vi "rosinterface-1.vi"() -> ()   [LabVIEW 2016]
uses:
  <userlib>/ROS for LabVIEW Software/ROS/Code/SubVIs/_ROSControl.ctl
  <userlib>/ROS for LabVIEW Software/ROS/Code/SubVIs/_ROSDirection.ctl
  <userlib>/ROS for LabVIEW Software/ROS/Code/Console/Servers/ServerSubs/TopicDef.ctl
  <userlib>/ROS for LabVIEW Software/ROS/MessageBuilding/std_msgs/subs/stringScalar.vi
  <userlib>/ROS for LabVIEW Software/ROS/MessageParsing/std_msgs/subs/parse_string_scalar.vi
panel:
  out "ROS out 2":T1={"topic port"=0, "Node"="", "topic"="", "type"="", "node port"=0, "error "={"status"=FALSE, "code"=0, "source"=""}, "Direction"=enum."Node", "Update (ms)"=1, "FIFO size"=1}
  in  "table 6":bool
  in  "table 5":bool
  in  "table 4":bool
  in  "table 3":bool
  in  "table2":bool
  in  "table 1":bool
  out "ROS out":T1={"topic port"=0, "Node"="", "topic"="", "type"="", "node port"=0, "error "={"status"=FALSE, "code"=0, "source"=""}, "Direction"=enum."Node", "Update (ms)"=1, "FIFO size"=1}
  in  "stop":bool
  out "Table  5":bool
  out "Table  4":bool
  out "Table  3":bool
  out "Table  2":bool
  out "Table 1":bool
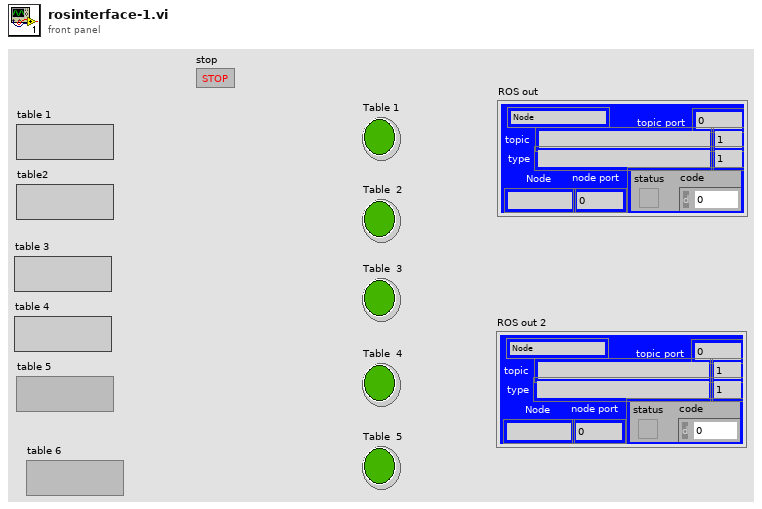
[diagram p1: front panel]
types:
  T1 = typedef "_ROSControl.ctl" = cluster{"topic port":u16, "Node":string, "topic":string, "type":string, "node port":u16, "error ":errorcluster, "Direction":T2, "Update (ms)":u16, "FIFO size":u16}
  T2 = typedef "_ROSDirection.ctl" = enum16{"Node", "Publisher", "Subscriber", "ServiceClient", "ServiceProvider"}
  T3 = typedef "TopicDef.ctl" = cluster{"Topic":string, "Type":string, "Action":T2, "Update (ms)":u16, "queue size":u16}
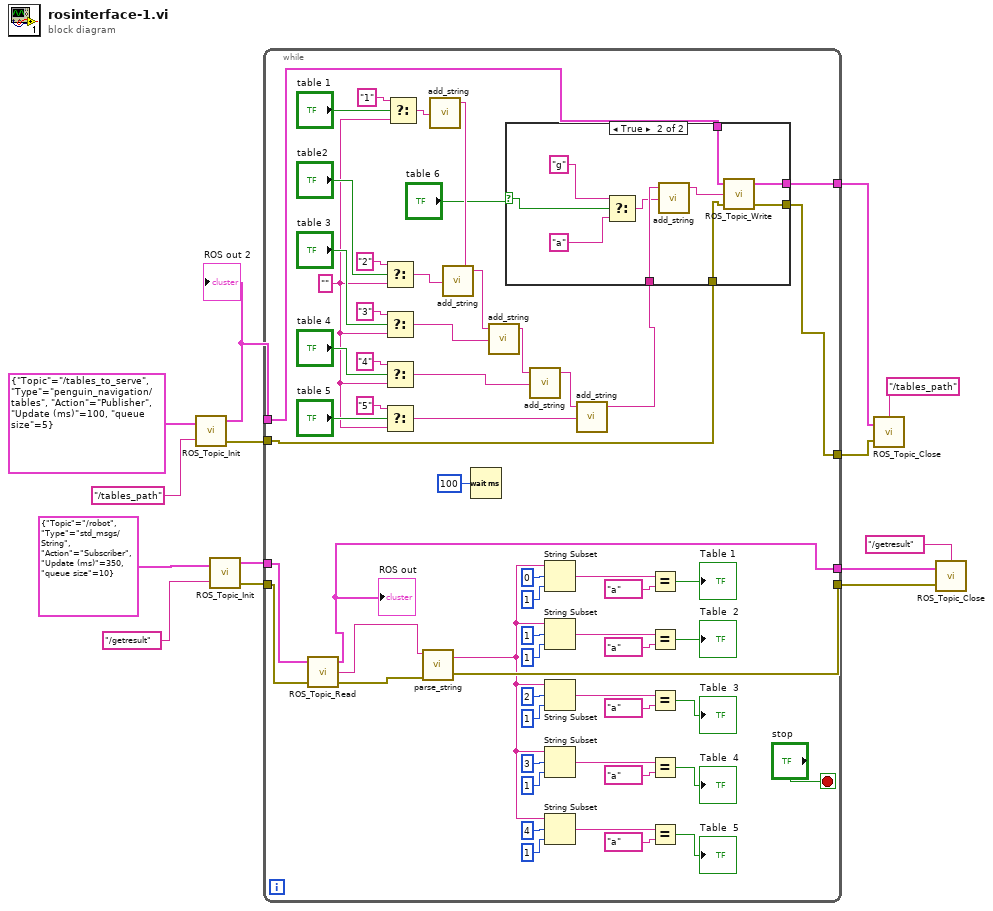
[diagram p0: block diagram]
diagram:
  n1 = call <userlib>:"ROS_Topic_Init.vi"("Definitions"=T3 {"Topic"="/tables_to_serve", "Type"="penguin_navigation/tables", "Action"=enum."Publisher", "Update (ms)"=100, "queue size"=5}, "node"="/tables_path") -> ("ROS out"=w8:T1, "error out"=w7:errorcluster)  [unwired: 1 in]
  "ROS out 2" <- w8
  n2 = call <userlib>:"ROS_Topic_Init.vi"("Definitions"=T3 {"Topic"="/robot", "Type"="std_msgs/String", "Action"=enum."Subscriber", "Update (ms)"=350, "queue size"=10}, "node"="/getresult") -> ("ROS out"=w4:T1, "error out"=w3:errorcluster)  [unwired: 1 in]
  n3 = while {
    tunnel: w4 -> [w28]
    tunnel: [w26] -> w13
    tunnel: w3 -> [w27]
    tunnel: [w74] -> w12
    tunnel: w8 -> [w19]
    tunnel: w7 -> [w18]
    tunnel: [w17] -> w2
    tunnel: [w16] -> w1
    stop <- "stop" stop-if-true
    w61 = "" ("t")
    n4 = call <userlib>:"ROS_Topic_Read.vi"("error in (no error)"=w27, "ROS in"=w28) -> ("error out"=w24:errorcluster, "Reply"=w25:string, "ROS out"=w26:T1)  [unwired: 1 in]
    "ROS out" <- w26
    n5 = Select(t="2", s="table2", f=w61) -> (s? t:f=w69:string)
    n6 = Select(t="3", s="table 3", f=w61) -> (s? t:f=w70:string)
    n7 = Select(t="4", s="table 4", f=w61) -> (s? t:f=w71:string)
    n8 = Select(t="5", s="table 5", f=w61) -> (s? t:f=w72:string)
    n9 = Select(t="1", s="table 1", f=w61) -> (s? t:f=w23:string)
    n10 = call-poly <userlib>:"parse_string.vi"("error in"=w24, "msg in"=w25) -> ("error out"=w74:errorcluster, "string"=w31:string)  [unwired: 3 in, 1 out]
    n11 = call-poly <userlib>:"add_string.vi"("String"=w23) -> ("msg out"=w22:string)  [unwired: 4 in]
    n12 = call-poly <userlib>:"add_string.vi"("String"=w69, "msg in"=w22) -> ("msg out"=w68:string)  [unwired: 3 in]
    n13 = Wait (ms)(milliseconds to wait=u32 100) -> ()  [unwired: 1 out]
    n14 = call-poly <userlib>:"add_string.vi"("String"=w70, "msg in"=w68) -> ("msg out"=w67:string)  [unwired: 3 in]
    n15 = call-poly <userlib>:"add_string.vi"("String"=w71, "msg in"=w67) -> ("msg out"=w73:string)  [unwired: 3 in]
    n16 = String Subset(string=w31, offset (0)=0, length (rest)=1 ("offset (0)")) -> (substring=w45:string)
    n17 = String Subset(string=w31, offset (0)=1, length (rest)=1 ("offset (0)")) -> (substring=w44:string)
    n18 = String Subset(string=w31, offset (0)=2, length (rest)=1 ("offset (0)")) -> (substring=w43:string)
    n19 = String Subset(string=w31, offset (0)=3, length (rest)=1 ("offset (0)")) -> (substring=w42:string)
    n20 = String Subset(string=w31, offset (0)=4, length (rest)=1 ("offset (0)")) -> (substring=w41:string)
    n21 = call-poly <userlib>:"add_string.vi"("String"=w72, "msg in"=w73) -> ("msg out"=w21:string)  [unwired: 3 in]
    n22 = case shown="True" "table 6" {
      selector: "table 6" -> [_ w80]
      tunnel: w21 -> [_ w82]
      tunnel: w19 -> [_ w78]
      tunnel: w18 -> [_ w77]
      tunnel: [_ w76] -> w17
      tunnel: [_ w75] -> w16
      frame False {
      }
      frame True {
        n23 = Select(t="g", s=w80, f="a") -> (s? t:f=w81:string)
        n24 = call-poly <userlib>:"add_string.vi"("String"=w81, "msg in"=w82) -> ("msg out"=w79:string)  [unwired: 3 in]
        n25 = call <userlib>:"ROS_Topic_Write.vi"("error in (no error)"=w77, "Msg in"=w79, "ROS in"=w78) -> ("error out"=w76:errorcluster, "ROS out"=w75:T1)  [unwired: 1 in]
      }
    }
    n26 = Equal?(x=w45, y="a") -> (x = y?=→"Table 1":bool)
    n27 = Equal?(x=w44, y="a") -> (x = y?=→"Table  2":bool)
    n28 = Equal?(x=w43, y="a") -> (x = y?=→"Table  3":bool)
    n29 = Equal?(x=w42, y="a") -> (x = y?=→"Table  4":bool)
    n30 = Equal?(x=w41, y="a") -> (x = y?=→"Table  5":bool)
  }
  n31 = call <userlib>:"ROS_Topic_Close.vi"("error in"=w2, "ROS in"=w1, "node"="/tables_path") -> ()  [unwired: 1 in, 1 out]
  n32 = call <userlib>:"ROS_Topic_Close.vi"("error in"=w12, "ROS in"=w13, "node"="/getresult") -> ()  [unwired: 1 in, 1 out]
